vi "ADO Recordset Destroy.vi"(8 "error in (no error)":errorcluster, 11 "ADODB._Recordset In":refnum<k7>) -> (0 "error out":errorcluster)   [LabVIEW 2013]
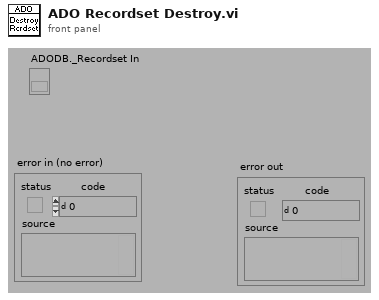
[diagram p1: front panel]
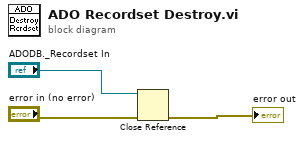
[diagram p0: block diagram]
diagram:
  n1 = Close Reference(reference="ADODB._Recordset In", error in (no error)="error in (no error)") -> (error out=→"error out":errorcluster)
